vi "Izhikevich_primitive_v007.vi"(0 "UDP Network Connection in":refnum<k16>, 1 "b":dbl, 2 "a":dbl, 3 "I":dbl, 5 "c":dbl, 7 "d":dbl, 9 "v(t)":dbl, 10 "Time":dbl, 11 "error in (no error)":errorcluster, 12 "u(t)":dbl, 13 "dt":dbl, 14 "Interval":dbl) -> (4 "UDP Network Connection out":refnum<k16>, 6 "v(t+dt)":dbl, 8 "u(t+dt)":dbl, 15 "error out":errorcluster)   [LabVIEW 2019]
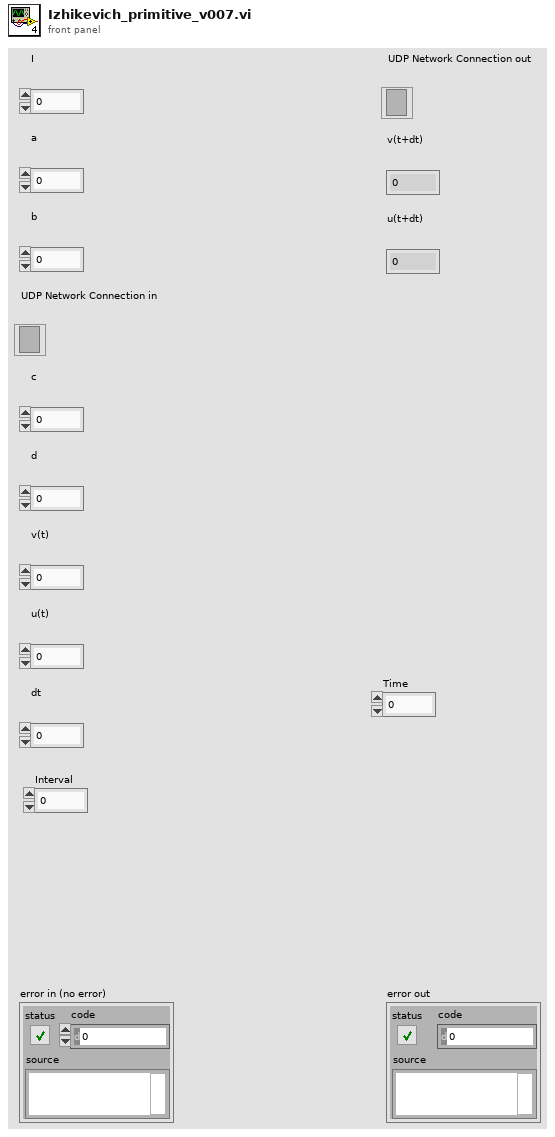
[diagram p1: front panel]
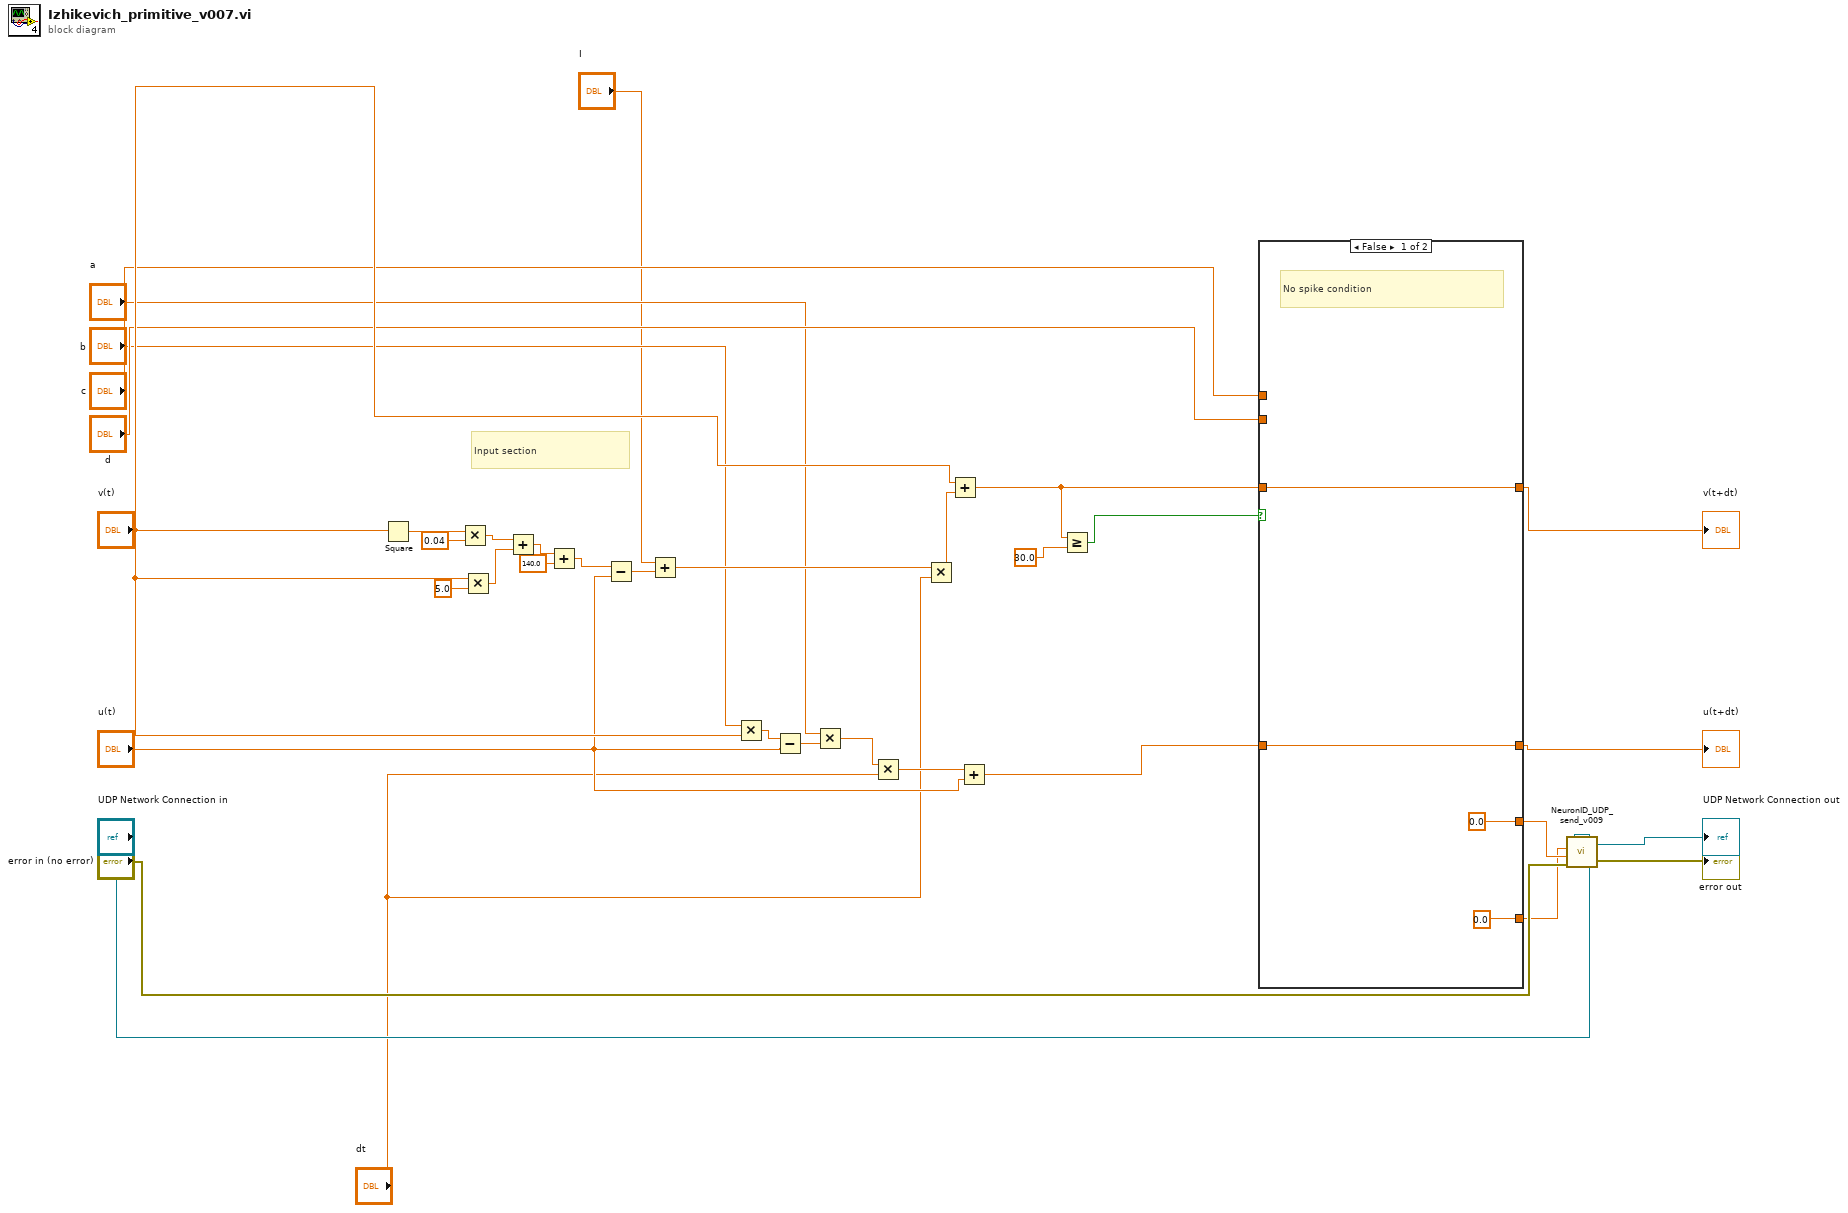
[diagram p0: block diagram]
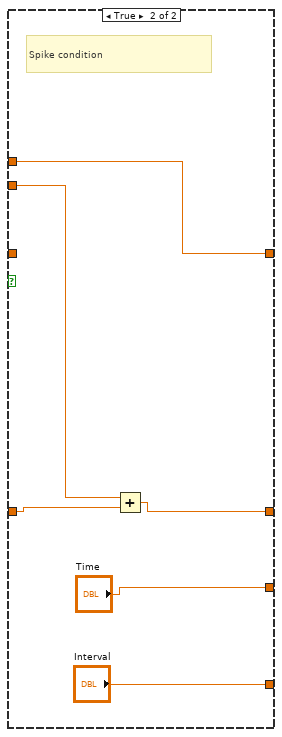
[diagram p2: hidden frame]
diagram:
  # "Input section"
  n1 = Square(x="v(t)") -> (x^2=w5:dbl)
  n2 = Multiply(x=w5, y=0.04) -> (x*y=w7:dbl)
  n3 = Multiply(x="v(t)", y=5.0) -> (x*y=w9:dbl)
  n4 = Add(x=w7, y=w9) -> (x+y=w10:dbl)
  n5 = Add(x=w10, y=140.0) -> (x+y=w12:dbl)
  n6 = Subtract(x=w12, y="u(t)") -> (x-y=w13:dbl)
  n7 = Add(x="I", y=w13) -> (x+y=w20:dbl)
  n8 = Multiply(x="b", y="v(t)") -> (x*y=w16:dbl)
  n9 = Subtract(x=w16, y="u(t)") -> (x-y=w17:dbl)
  n10 = Multiply(x="a", y=w17) -> (x*y=w19:dbl)
  n11 = Multiply(x=w19, y="dt") -> (x*y=w23:dbl)
  n12 = Multiply(x=w20, y="dt") -> (x*y=w22:dbl)
  n13 = Add(x="v(t)", y=w22) -> (x+y=w32:dbl)
  n14 = Add(x=w23, y="u(t)") -> (x+y=w25:dbl)
  n15 = Greater Or Equal?(x=w32, y=30.0) -> (x >= y?=w33:bool)
  n16 = case shown="False" w33 {
    tunnel: [w39 w42] -> w24
    tunnel: w25 -> [w39 w44]
    tunnel: w32 -> [w38 _]
    tunnel: [w38 w45] -> w26
    tunnel: "c" -> [_ w45]
    tunnel: "d" -> [_ w43]
    tunnel: [0.0 ("Neuron ID") "Time"] -> w4
    tunnel: [0.0 ("Neuron ID") "Interval"] -> w1
    frame False {
      # "No spike condition"
    }
    frame True {
      # "Spike condition"
      n17 = Add(x=w43, y=w44) -> (x+y=w42:dbl)
    }
  }
  "v(t+dt)" <- w26
  "u(t+dt)" <- w24
  n18 = call "NeuronID_UDP_send_v009.vi"("error in (no error)"="error in (no error)", "Neuron ID"=w4, "Interval"=w1, "UDP Network Connection in"="UDP Network Connection in") -> ("error out"=→"error out":errorcluster, "UDP Network Connection out"=→"UDP Network Connection out":refnum<k16>)
